vi "Send Set Start Parameter.vi"(7 "Message Priority (Normal)":T3=enum."Normal", 8 "error in (no error)":errorcluster, 10 "Start Parameter":T1={"Windows Titel"="", "Start WorkDir"=path "C:/Users/user/Desktop/test/WorkDir", "Camera ConfigDir"=path "C:/Users/user/Desktop/test/ConfigDir", "Camera"="TestCam", "OverlayColor"=13816530, "TimeInFilename"=FALSE, "TimestampFormat"="%H.%M.%S%3u", "ShotIdInFilename"=FALSE, "CamInFilename"=FALSE}, 11 "Message Enqueuer":refnum<class "Message Enqueuer.lvclass">) -> (0 "error out":errorcluster, 3 "Message Enqueuer out":refnum<class "Message Enqueuer.lvclass">)   [LabVIEW 2020, in "HIJ Vision Launcher.lvlib" / "Set Start Parameter Msg.lvclass"]
doc: "This VI sends the message to an actor."
uses:
  Set Start Parameter Msg.lvclass
  <vilib>/ActorFramework/Message Enqueuer/Message Enqueuer.lvclass
  <vilib>/ActorFramework/Message Enqueuer/Message Priority.ctl
  HIJ Vision Launcher/Start Parameter.ctl
  <vilib>/userdefined/High Color/IMAQdx.ctl
  C:/Program Files (x86)/National Instruments/LabVIEW 2020/vi.lib/ActorFramework/Message/Message.lvclass
  Set Start Parameter Msg.lvclass/Set Start Parameter Msg.ctl
  <vilib>/ActorFramework/Message Enqueuer/Message Enqueuer.lvclass/Message Enqueuer.ctl
  <vilib>/ActorFramework/Message Priority Queue/Priority Enqueue.vi
  HIJ Vision Launcher/HIJ Vision Launcher.lvclass
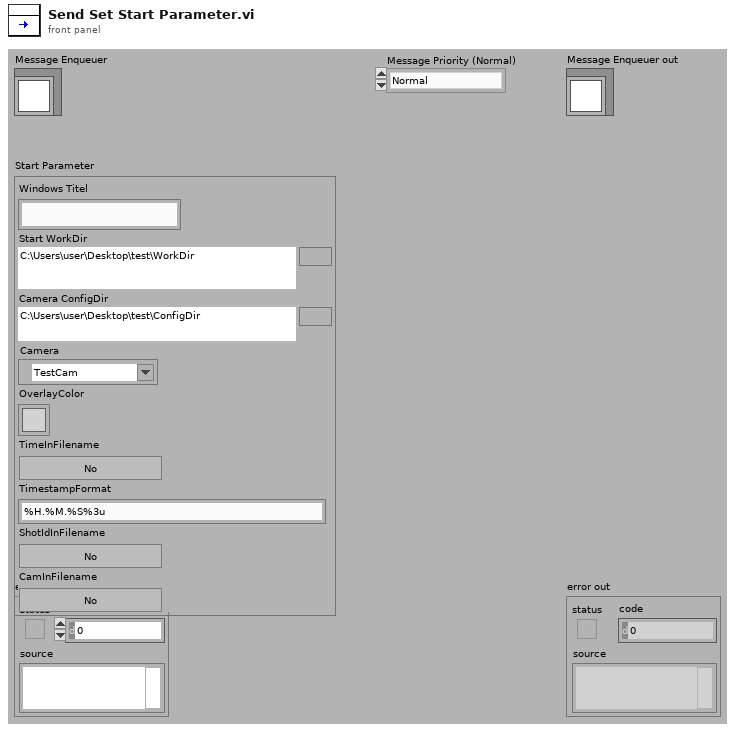
[diagram p1: front panel]
types:
  T1 = typedef "HIJ Vision Launcher.lvlib/HIJ Vision Launcher.lvclass/Start Parameter.ctl" = cluster{"Windows Titel":string, "Start WorkDir":path, "Camera ConfigDir":path, "Camera":T2, "OverlayColor":u32, "TimeInFilename":bool, "TimestampFormat":string, "ShotIdInFilename":bool, "CamInFilename":bool}
  T2 = typedef "IMAQdx.ctl" = refnum<k21>
  T3 = typedef "Actor Framework.lvlib/Message Enqueuer.lvclass/Message Priority.ctl" = enum16{"Low", "Normal", "High"}
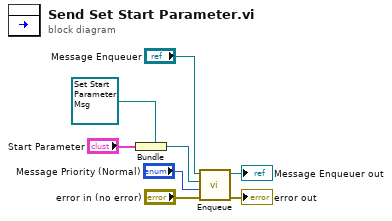
[diagram p0: block diagram]
diagram:
  n1 = Bundle(cluster=refnum<class "Set Start Parameter Msg.lvclass"> refnum ("Object"), "Start Parameter") -> (w4:refnum<class "Set Start Parameter Msg.lvclass">)
  n2 = call <vilib>:"Enqueue.vi"("error in (no error)"="error in (no error)", "Message Priority (Normal)"="Message Priority (Normal)", "Message"=w4, "Message Enqueuer in"="Message Enqueuer") -> ("error out"=→"error out":errorcluster, "Message Enqueuer out"=→"Message Enqueuer out":refnum<class "Message Enqueuer.lvclass">)  [unwired: 6 in]
